vi "SmoothMovePane.vi"(8 "error in (no error)":errorcluster, 10 "Origin":T1, 11 "Pane in":refnum<vi>) -> (0 "error out":errorcluster)   [LabVIEW 2012, in "Win8uiFramework.lvlib" / "MainController.lvclass"]
uses:
  MainController.lvclass
  <vilib>/Utility/miscctls.llb/LVPointTypeDef.ctl
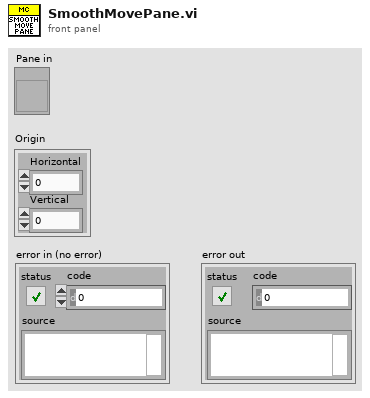
[diagram p1: front panel]
types:
  T1 = typedef "LVPointTypeDef.ctl" = cluster{"Horizontal":i16, "Vertical":i16}
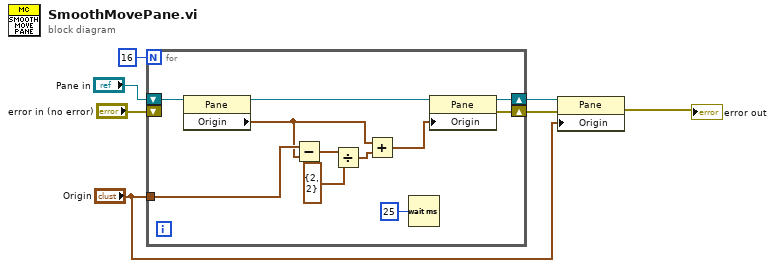
[diagram p0: block diagram]
diagram:
  n1 = for {
    N: 16 -> [_]
    tunnel: "Origin" -> [w15]
    shift-right: [w18] -> w3
    shift-left: "error in (no error)" -> [_]
    shift-right: [w8] -> w4
    shift-left: "Pane in" -> [w17]
    n2 = property class="Pane"(reference=w17) -> (reference out=w16:refnum<vi>, "Origin"=w11:T1)  [unwired: 1 in, 1 out]
    n3 = Subtract(x=w15, y=w11) -> (x-y=w14:T1)
    n4 = Divide(x=w14, y=T1 {"Horizontal"=2, "Vertical"=2}) -> (x/y=w12:cluster{"Horizontal":dbl, "Vertical":dbl})
    n5 = Add(x=w11, y=w12) -> (x+y=w10:cluster{"Horizontal":dbl, "Vertical":dbl})
    n6 = Wait (ms)(milliseconds to wait=u32 25) -> ()  [unwired: 1 out]
    n7 = property class="Pane"(reference=w16, "Origin"=w10) -> (reference out=w8:refnum<vi>, error out=w18:errorcluster)  [unwired: 1 in]
  }
  n8 = property class="Pane"(reference=w4, error in=w3, "Origin"="Origin") -> (error out=→"error out":errorcluster)  [unwired: 1 out]
